vi "save echarpe image.vi"() -> ()   [LabVIEW 2018]
uses:
  RxTx/RxTx.lvclass
  Save Image/Save Image.lvclass
  Python Toolkit/Python Toolkit.lvclass/Python Toolkit.ctl
  Channel/Channel.lvclass
  Python Toolkit/Python Toolkit.lvclass
panel:
  in  "Save Image.lvclass":refnum<class "Save Image.lvclass">
  in  "Stop Button":bool
  out "error out":errorcluster
  in  "RxTx.lvclass":refnum<class "RxTx.lvclass">
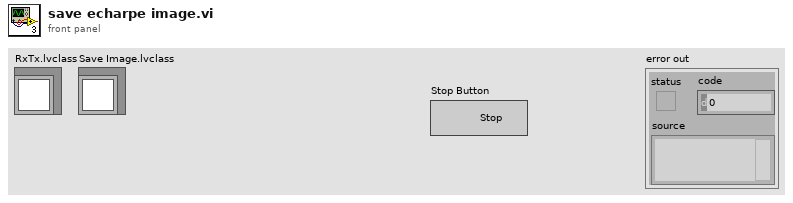
[diagram p1: front panel]
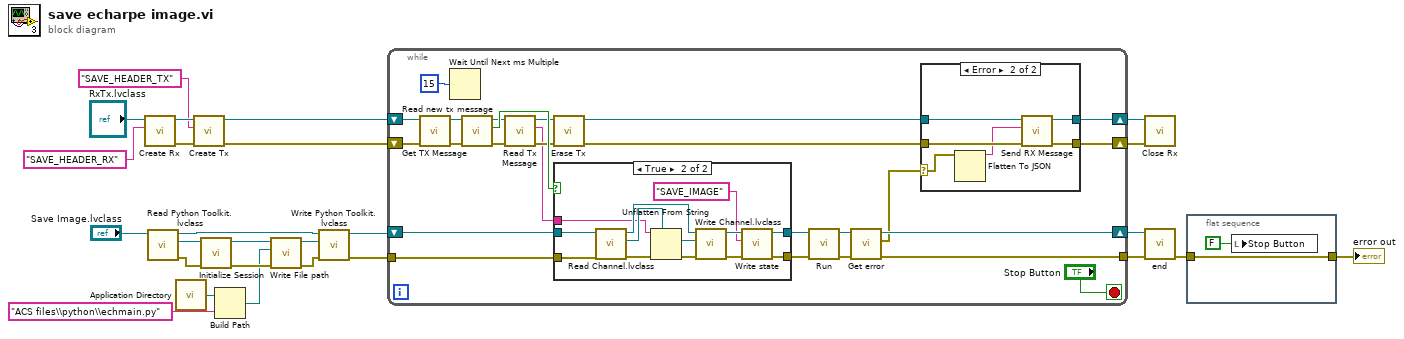
[diagram p0: block diagram]
diagram:
  n1 = call "Create Rx.vi"("Reader Name"="SAVE_HEADER_RX", "RxTx in"="RxTx.lvclass") -> ("error out"=w22:errorcluster, "RxTx out"=w23:refnum<class "RxTx.lvclass">)  [unwired: 8 in]
  n2 = call-dynamic "Read Python Toolkit.lvclass.vi"("Save Image in"="Save Image.lvclass") -> ("error out"=w9:errorcluster, "Python Toolkit.lvclass"=w8:refnum<class "Python Toolkit.lvclass">, "Save Image out"=w4:refnum<class "Save Image.lvclass">)  [unwired: 8 in]
  n3 = call <vilib>:"Application Directory.vi"() -> ("Application Directory"=w12:path)
  n4 = call "Create Tx.vi"("error in (no error)"=w22, "Writer Name"="SAVE_HEADER_TX" ("Reader Name"), "RxTx in"=w23) -> ("error out"=w16:errorcluster, "RxTx out"=w17:refnum<class "RxTx.lvclass">)  [unwired: 7 in]
  n5 = call "Initialize Session.vi"("error in (no error)"=w9, "Python Toolkit in"=w8) -> ("error out"=w13:errorcluster, "Python Toolkit out"=w7:refnum<class "Python Toolkit.lvclass">)  [unwired: 8 in]
  n6 = Build Path(base path=w12, name or relative path="ACS files\\python\\echmain.py") -> (appended path=w10:path)
  n7 = call "Write File path.vi"("error in (no error)"=w13, "File path"=w10, "Python Toolkit in"=w7) -> ("error out"=w5:errorcluster, "Python Toolkit out"=w6:refnum<class "Python Toolkit.lvclass">)  [unwired: 7 in]
  n8 = call-dynamic "Write Python Toolkit.lvclass.vi"("error in (no error)"=w5, "Python Toolkit.lvclass"=w6, "Save Image in"=w4) -> ("error out"=w2:errorcluster, "Save Image out"=w3:refnum<class "Save Image.lvclass">)  [unwired: 7 in]
  n9 = while {
    shift-right: [w30] -> w20
    shift-left: w17 -> [w41]
    shift-right: [w44] -> w24
    shift-left: w3 -> [w48]
    shift-right: [w29] -> w18
    shift-left: w16 -> [w42]
    tunnel: [w45] -> w19
    tunnel: w2 -> [w27]
    stop <- "Stop Button" stop-if-true
    n10 = call "Get TX Message.vi"("error in (no error)"=w42, "RxTx in"=w41) -> ("error out"=w40:errorcluster, "RxTx out"=w39:refnum<class "RxTx.lvclass">)  [unwired: 8 in]
    n11 = Wait Until Next ms Multiple(millisecond multiple=u32 15) -> ()  [unwired: 1 out]
    n12 = call-dynamic "Read new tx message.vi"("error in (no error)"=w40, "RxTx in"=w39) -> ("error out"=w37:errorcluster, "new tx message"=w38:bool, "RxTx out"=w34:refnum<class "RxTx.lvclass">)  [unwired: 7 in]
    n13 = call "Read Tx Message.vi"("error in (no error)"=w37, "RxTx in"=w34) -> ("error out"=w36:errorcluster, "Tx Message"=w33:string, "RxTx out"=w35:refnum<class "RxTx.lvclass">)  [unwired: 7 in]
    n14 = call "Erase Tx.vi"("error in (no error)"=w36, "RxTx in"=w35) -> ("error out"=w31:errorcluster, "RxTx out"=w32:refnum<class "RxTx.lvclass">)  [unwired: 8 in]
    n15 = case shown="True" w38 {
      tunnel: [w61 w67] -> w50
      tunnel: [w60 w65] -> w49
      tunnel: w48 -> [w61 w74]
      tunnel: w33 -> [_ w63]
      tunnel: w27 -> [w60 w62]
      frame False {
      }
      frame True, Default {
        n16 = call "Read Channel.lvclass.vi"("error in (no error)"=w62, "Save Image in"=w74) -> ("error out"=w73:errorcluster, "Channel.lvclass"=w70:refnum<class "Channel.lvclass">, "Save Image out"=w71:refnum<class "Save Image.lvclass">)  [unwired: 7 in]
        n17 = Unflatten From String(type=w70, binary string=w63, error in (no error)=w73) -> (value=w69:refnum<class "Channel.lvclass">, error out=w72:errorcluster)  [unwired: 2 in, 1 out]
        n18 = call-dynamic "Write Channel.lvclass.vi"("error in (no error)"=w72, "Channel.lvclass"=w69, "Save Image in"=w71) -> ("error out"=w66:errorcluster, "Save Image out"=w68:refnum<class "Save Image.lvclass">)  [unwired: 7 in]
        n19 = call "Write state.vi"("error in (no error)"=w66, "String"="SAVE_IMAGE" ("Reader Name"), "Save Image in"=w68) -> ("error out"=w65:errorcluster, "Save Image out"=w67:refnum<class "Save Image.lvclass">)  [unwired: 7 in]
      }
    }
    n20 = call-dynamic "Run.vi"("error in (no error)"=w49, "Save Image in"=w50) -> ("error out"=w46:errorcluster, "Save Image out"=w43:refnum<class "Save Image.lvclass">)  [unwired: 8 in]
    n21 = call "Get error.vi"("error in (no error)"=w46, "Save Image in"=w43) -> ("error out"=w45:errorcluster, "error"=w28:errorcluster, "Save Image out"=w44:refnum<class "Save Image.lvclass">)  [unwired: 7 in]
    n22 = case shown="Error" w28 {
      selector: w28 -> [_ w55]
      tunnel: w32 -> [w53 w59]
      tunnel: w31 -> [w52 w56]
      tunnel: [w53 w58] -> w30
      tunnel: [w52 w57] -> w29
      frame No Error {
      }
      frame Error {
        n23 = Flatten To JSON(anything=w55) -> (JSON string=w54:string)  [unwired: 2 in, 1 out]
        n24 = call "Send RX Message.vi"("error in (no error)"=w56, "element"=w54, "RxTx in"=w59) -> ("error out"=w57:errorcluster, "RxTx out"=w58:refnum<class "RxTx.lvclass">)  [unwired: 7 in]
      }
    }
  }
  n25 = call "Close Rx.vi"("error in (no error)"=w18, "RxTx in"=w20) -> ()  [unwired: 8 in, 2 out]
  n26 = call "end.vi"("error in (no error)"=w19, "Save Image in"=w24) -> ("error out"=w15:errorcluster)  [unwired: 8 in, 1 out]
  n27 = flat-sequence {
    tunnel: w15 -> [w76]
    tunnel: [w76] -> w14
    frame #0 {
      n28 = local write "Stop Button"(FALSE ("Stop Button")) -> ()
    }
  }
  "error out" <- w14
